vi "FTS GetSet Acquisition Option PD tempCtrl.vi"(6 "read/write":enum16{"read", "write"}(ring), 7 "PD sensitivity mode Pre":T1, 8 "error in":errorcluster, 9 "PD sensitivity mode write":T1, 10 "channel index interferogram":u16, 11 "spectrometerIdx":u16) -> (0 "error out":errorcluster, 1 "PD sensitivity mode out":T1, 3 "status FTSLib":i32)   [LabVIEW 2010, in "FTSLib.lvlib"]
uses:
  FTSLib.lvlib
  _misc/Thorlabs_FTS_misc.llb/PDTemperatureMode.ctl
  FTSLib.dll
  OSA20X_misc.lvlib
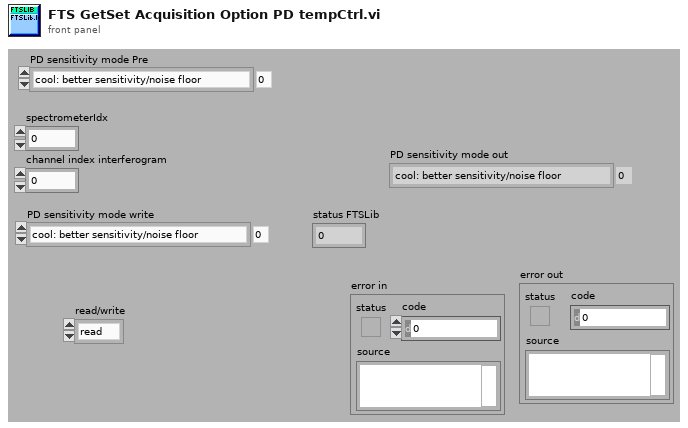
[diagram p1: front panel]
types:
  T1 = typedef "OSA20X_misc.lvlib/PDTemperatureMode.ctl" = enum16{"cool: better sensitivity/noise floor", "warm: extended wl range"}
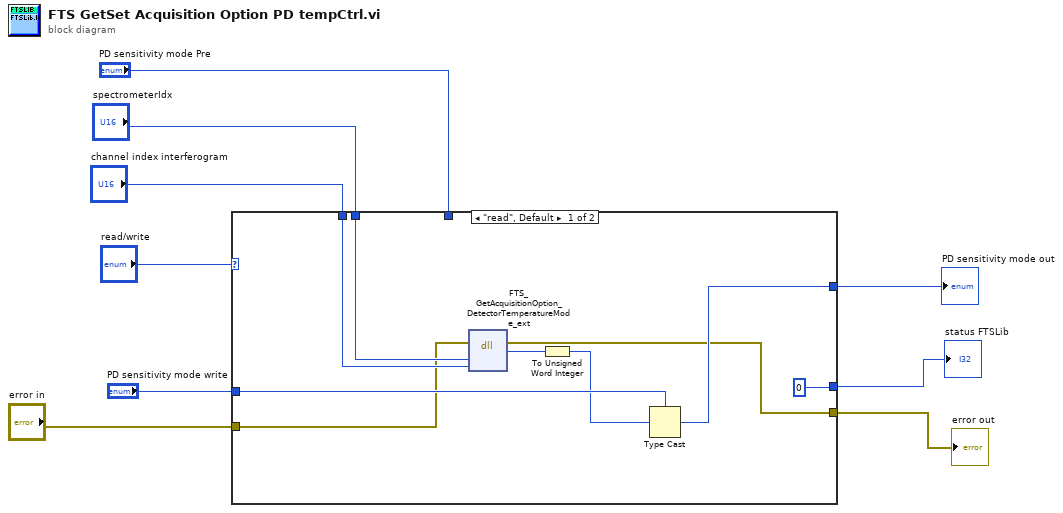
[diagram p0: block diagram]
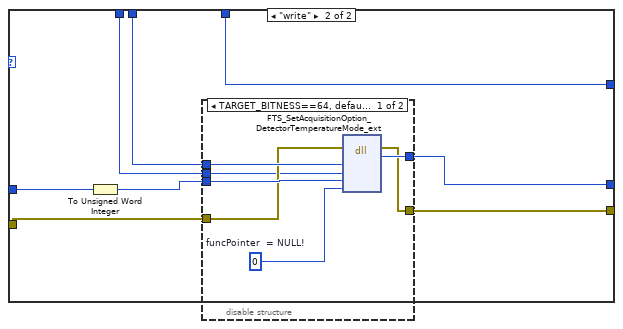
[diagram p2: hidden frame]
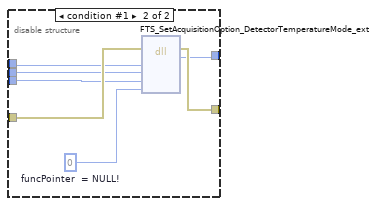
[diagram p3: hidden frame]
diagram:
  n1 = case shown="\"read\", Default" "read/write" {
    tunnel: "error in" -> [w10 w24]
    tunnel: [w13 w21] -> w5
    tunnel: "PD sensitivity mode write" -> [w16 w20]
    tunnel: [0 ("return type") w22] -> w3
    tunnel: "spectrometerIdx" -> [w18 w26]
    tunnel: [w14 w19] -> w2
    tunnel: "channel index interferogram" -> [w12 w23]
    tunnel: "PD sensitivity mode Pre" -> [_ w19]
    frame "read", Default {
      n2 = dll-call lib="FTSLib.dll" fn="FTS_GetAcquisitionOption_DetectorTemperatureMode_ext"(error in=w10, "spectrIdx"=w18, "channel"=w12) -> (error out=w13:errorcluster, "return type"=w17:i32)  [unwired: 4 in, 1 out]
      n3 = To Unsigned Word Integer(number=w17) -> (unsigned 16bit integer=w15:u16)
      n4 = Type Cast(type=w16, x=w15) -> (*(type *) &x=w14:T1)
    }
    frame "write" {
      n5 = To Unsigned Word Integer(number=w20) -> (unsigned 16bit integer=w25:u16)
      n6 = disable-structure shown="TARGET_BITNESS==64, default" {
        disable-tunnel: [w33 w35] -> w22
        disable-tunnel: w26 -> [w32 w37]
        disable-tunnel: w25 -> [w30 w36]
        disable-tunnel: w24 -> [w29 w39]
        disable-tunnel: [w28 w38] -> w21
        disable-tunnel: w23 -> [w27 w34]
        frame condition #0 (active) {
          w31 = u64 0  # funcPointer  = NULL!
          n7 = dll-call lib="FTSLib.dll" fn="FTS_SetAcquisitionOption_DetectorTemperatureMode_ext"(error in=w29, "spectrIdx"=w32, "channel"=w27, "sensitivityMode"=w30, "funcPointer"=w31) -> (error out=w28:errorcluster, "return type"=w33:i32)  [unwired: 6 in, 1 out]
        }
        frame condition #1 {
          w40 = u32 0  # funcPointer  = NULL!
          n8 = dll-call lib="FTSLib.dll" fn="FTS_SetAcquisitionOption_DetectorTemperatureMode_ext"(error in=w39, "spectrIdx"=w37, "channel"=w34, "sensitivityMode"=w36, "funcPointer"=w40) -> (error out=w38:errorcluster, "return type"=w35:i32)  [unwired: 6 in, 1 out]
        }
      }
    }
  }
  "error out" <- w5
  "status FTSLib" <- w3
  "PD sensitivity mode out" <- w2
